vi "SortIVTraces.vi"(10 "Array in":waveform(dbl)[](array[waveform]), 11 "Waveform":waveform(dbl)) -> (1 "Array 6":cluster{"Y":dbl[], "Y":dbl[]}[](array[cluster]), 2 "Array 3":cluster{"Y":dbl[], "Y":dbl[]}[](array[cluster]), 3 "Array out":string[][](array[string]), 4 "Array 4":cluster{"Y":dbl[], "Y":dbl[]}[](array[cluster]), 5 "Array 5":cluster{"Y":dbl[], "Y":dbl[]}[](array[cluster]))   [LabVIEW 2024]
uses:
  2e77fa2f-ae95-4288-bad6-8e3e04a47533.vi
  <vilib>/Comparison/Less/Less Functor/Less Functor.lvclass
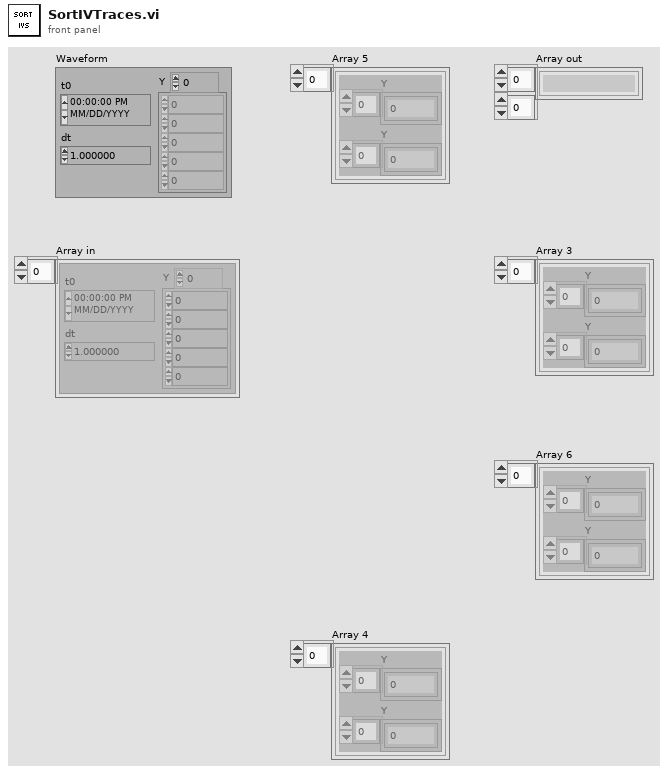
[diagram p1: front panel]
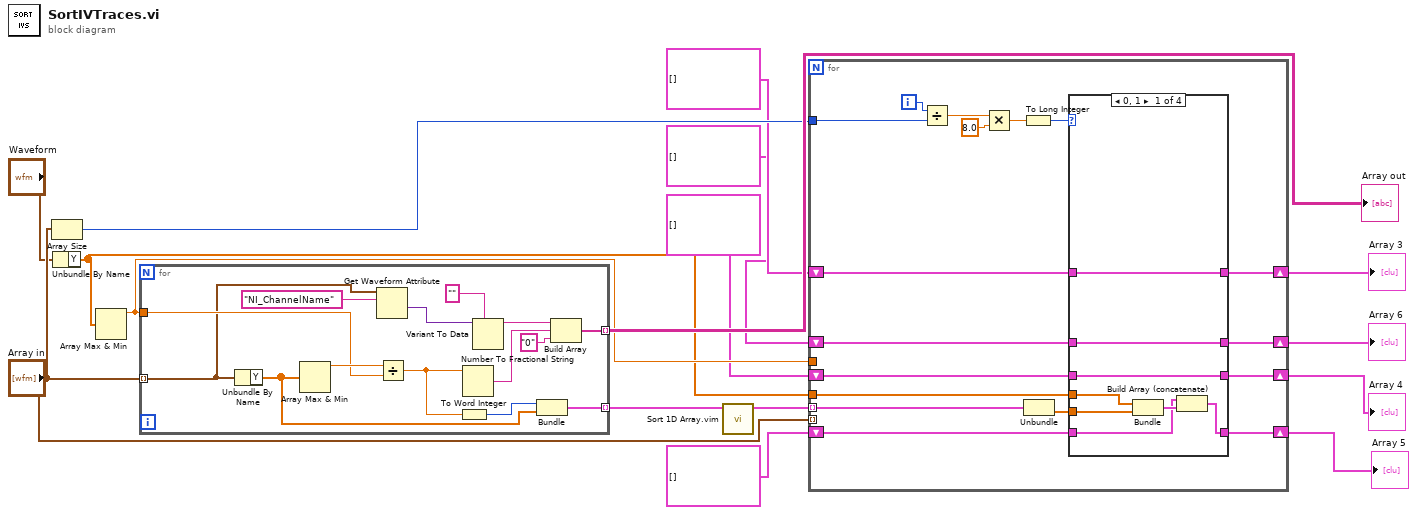
[diagram p0: block diagram]
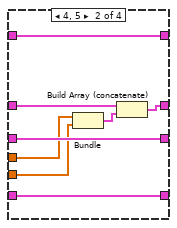
[diagram p2: hidden frame]
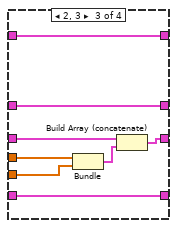
[diagram p3: hidden frame]
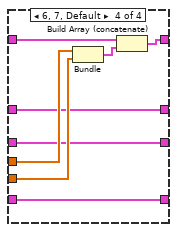
[diagram p4: hidden frame]
diagram:
  n1 = Array Size(array="Array in") -> (size(s)=w15:i32)
  n2 = Unbundle By Name("Waveform") -> ("Y"=w7:dbl[])
  n3 = Array Max & Min(array=w7) -> (max value=w11:dbl)  [unwired: 3 out]
  n4 = for {
    tunnel: "Array in" -> [w24] mode=indexing
    tunnel: w11 -> [w29]
    tunnel: [w26] -> w12 mode=indexing
    tunnel: [w19] -> w16 mode=indexing
    n5 = Unbundle By Name(w24) -> ("Y"=w27:dbl[])
    n6 = Array Max & Min(array=w27) -> (max value=w30:dbl)  [unwired: 3 out]
    n7 = Get Waveform Attribute(6:"NI_ChannelName" ("name"), 7:w24) -> (1:w23:variant)  [unwired: 2 in, 3 out]
    n8 = Divide(x=w30, y=w29) -> (x/y=w20:dbl)
    n9 = To Word Integer(number=w20) -> (16bit integer=w28:i16)
    n10 = Number To Fractional String(number=w20) -> (F-format string=w18:string)  [unwired: 3 in]
    n11 = Variant To Data(type="", Variant=w23) -> (data=w21:string)  [unwired: 1 in, 1 out]
    n12 = Bundle(w28, "Y"=w27) -> (w26:cluster{i16, "Y":dbl[]})  [unwired: 1 in]
    n13 = Build Array(w21, w18, "0" ("element")) -> (w19:string[])
  }
  "Array out" <- w16
  n14 = call "Sort 1D Array.vim"("unsorted array"=w12) -> ("sorted array"=w13:cluster{i16, "Y":dbl[]}[])  [unwired: 10 in]
  n15 = for {
    tunnel: "Array in" -> [_] mode=indexing
    shift-right: [w41] -> w10
    shift-left: cluster{"Y":dbl[], "Y":dbl[]}[] [] -> [w40]
    shift-right: [w44] -> w9
    shift-left: cluster{"Y":dbl[], "Y":dbl[]}[] [] -> [w45]
    shift-right: [w43] -> w6
    shift-left: cluster{"Y":dbl[], "Y":dbl[]}[] [] -> [w42]
    shift-right: [w46] -> w8
    shift-left: cluster{"Y":dbl[], "Y":dbl[]}[] [] -> [w47]
    tunnel: w7 -> [w39]
    tunnel: w11 -> [_]
    tunnel: w13 -> [w38] mode=indexing
    tunnel: w15 -> [w34]
    i -> [w36]
    n16 = Divide(x=w36, y=w34) -> (x/y=w35:dbl)
    n17 = Multiply(x=w35, y=8.0) -> (x*y=w33:dbl)
    n18 = To Long Integer(number=w33) -> (32bit integer=w31:i32)
    n19 = Unbundle(w38) -> ("Y"=w37:dbl[])  [unwired: 1 out]
    n20 = case shown="0, 1" w31 {
      tunnel: w47 -> [w52 w61 w66 w74]
      tunnel: w39 -> [w55 w58 w70 w78]
      tunnel: w37 -> [w54 w57 w69 w77]
      tunnel: [w51 w61 w66 w74] -> w46
      tunnel: w45 -> [w50 w60 w68 w73]
      tunnel: [w50 w60 w67 w73] -> w44
      tunnel: [w49 w62 w65 w72] -> w43
      tunnel: w42 -> [w49 w59 w65 w72]
      tunnel: [w48 w56 w64 w75] -> w41
      tunnel: w40 -> [w48 w56 w64 w76]
      frame 0, 1 {
        n21 = Bundle("Y"=w55, "Y"=w54) -> (w53:cluster{"Y":dbl[], "Y":dbl[]})  [unwired: 1 in]
        n22 = Build Array (concatenate)(w52, w53) -> (w51:cluster{"Y":dbl[], "Y":dbl[]}[])
      }
      frame 4, 5 {
        n23 = Bundle("Y"=w58, "Y"=w57) -> (w63:cluster{"Y":dbl[], "Y":dbl[]})  [unwired: 1 in]
        n24 = Build Array (concatenate)(w59, w63) -> (w62:cluster{"Y":dbl[], "Y":dbl[]}[])
      }
      frame 2, 3 {
        n25 = Bundle("Y"=w70, "Y"=w69) -> (w71:cluster{"Y":dbl[], "Y":dbl[]})  [unwired: 1 in]
        n26 = Build Array (concatenate)(w68, w71) -> (w67:cluster{"Y":dbl[], "Y":dbl[]}[])
      }
      frame 6, 7, Default {
        n27 = Bundle("Y"=w78, "Y"=w77) -> (w79:cluster{"Y":dbl[], "Y":dbl[]})  [unwired: 1 in]
        n28 = Build Array (concatenate)(w76, w79) -> (w75:cluster{"Y":dbl[], "Y":dbl[]}[])
      }
    }
  }
  "Array 3" <- w10
  "Array 4" <- w9
  "Array 5" <- w8
  "Array 6" <- w6
